vi "FT_Open_Device_By_Index_64bit.vi"(7 "error in (no error)":errorcluster, 10 "Device Index":u32) -> (0 "error out":errorcluster, 2 "FT_Status":u32(ring) items=["FT_OK", "FT_INVALID_HANDLE", "FT_DEVICE_NOT_FOUND", "FT_DEVICE_NOT_OPENED", "FT_IO_ERROR", "FT_INSUFFICIENT_RESOURCES", "FT_INVALID_PARAMETER", "FT_INVALID_BAUD_RATE", "FT_DEVICE_NOT_OPENED_FOR_ERASE", "FT_DEVICE_NOT_OPENED_FOR_WRITE", "FT_FAILED_TO_WRITE_DEVICE", "FT_EEPROM_READ_FAILED", "FT_EEPROM_WRITE_FAILED", "FT_EEPROM_ERASE_FAILED", "FT_EEPROM_NOT_PRESENT", "FT_EEPROM_NOT_PROGRAMMED", "FT_INVALID_ARGS", "FT_NOT_SUPPORTED", "FT_OTHER_ERROR"], 3 "Handle":u64)   [LabVIEW 2019]
uses:
  FTD2XX.dll
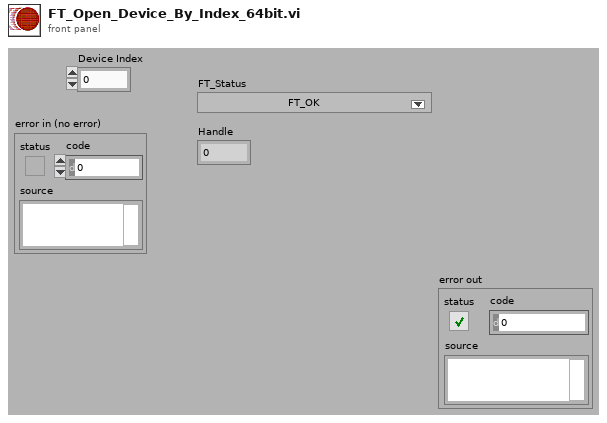
[diagram p1: front panel]
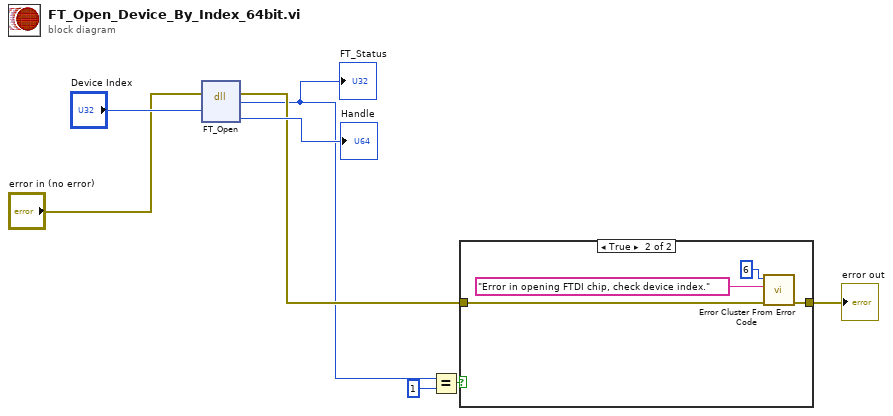
[diagram p0: block diagram]
diagram:
  n1 = dll-call lib="FTD2XX.dll" fn="FT_Open"(error in="error in (no error)", "DeviceIndex"="Device Index") -> (error out=w4:errorcluster, "FT_Status"=w2:u32, "Handle"=→"Handle":u64)  [unwired: 4 in, 1 out]
  "FT_Status" <- w2
  n2 = Equal?(x=w2, y=u32 1) -> (x = y?=w3:bool)
  n3 = case shown="True" w3 {
    tunnel: [w9 w12] -> w6
    tunnel: w4 -> [w9 w11]
    frame False {
    }
    frame True {
      n4 = call <vilib>:"Error Cluster From Error Code.vi"("error in (no error)"=w11, "error message (\"\")"="Error in opening FTDI chip, check device index." ("error message (\"\")"), "error code (0)"=6) -> ("error out"=w12:errorcluster)  [unwired: 6 in]
    }
  }
  "error out" <- w6
